vi "JL_Cycle_History_ParseRecord.vi"(5 "Low Level Tries":u8=5, 7 "Error In":errorcluster, 8 "Cycle History ERD":T1={"ERD Number"=61790, "Data Type"=enum."string"} {"ERD Number" format="%.0x"}, 9 "GEA Inputs":T2={"Source"=228, "Destination"=36} {"Destination" format="%.0x"; "Source" format="%.0x"}, 10 "GEA2 Reference In":refnum<k24>) -> (0 "Error Out":errorcluster, 1 "Bits":i32, 2 "CS2 Dryer":string[](array[string]), 3 "GEA2 Reference Out":refnum<k24>)   [LabVIEW 2023]
uses:
  D:/Common/LabVIEW GEA2 Toolkit/source/GEA3 DLL Source/GeaCommunication.dll
  Common/LabVIEW GEA2 Toolkit/source/GEA3 DLL Source/GeaCommunication.dll
  Common/LabVIEW GEA2 Toolkit/GEA3/type defs/Source_Destination.ctl
  Common/LabVIEW GEA2 Toolkit/GEA3/type defs/ERD Read Data In.ctl
  Common/LabVIEW GEA2 Toolkit/GEA3/library/GEA2_Toolkit.lvlib
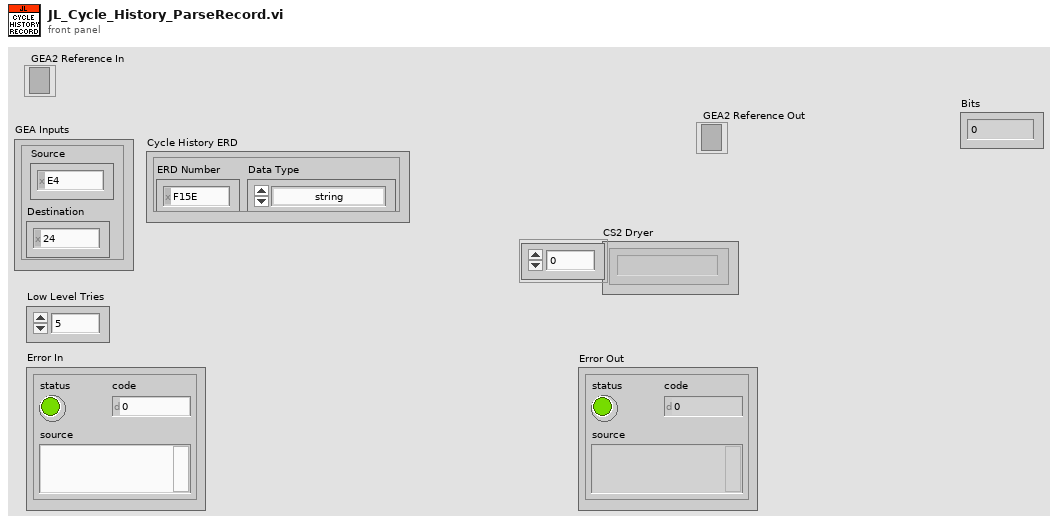
[diagram p1: front panel]
types:
  T1 = typedef "ERD Read Data In.ctl" = cluster{"ERD Number":u16, "Data Type":enum16{"string", "boolean", "uint8_t", "uint16_t", "uint32_t", "uint64_t", "int8_t", "int16_t", "int32_t", "int64_t"}}
  T2 = typedef "Source_Destination.ctl" = cluster{"Source":u8, "Destination":u8}
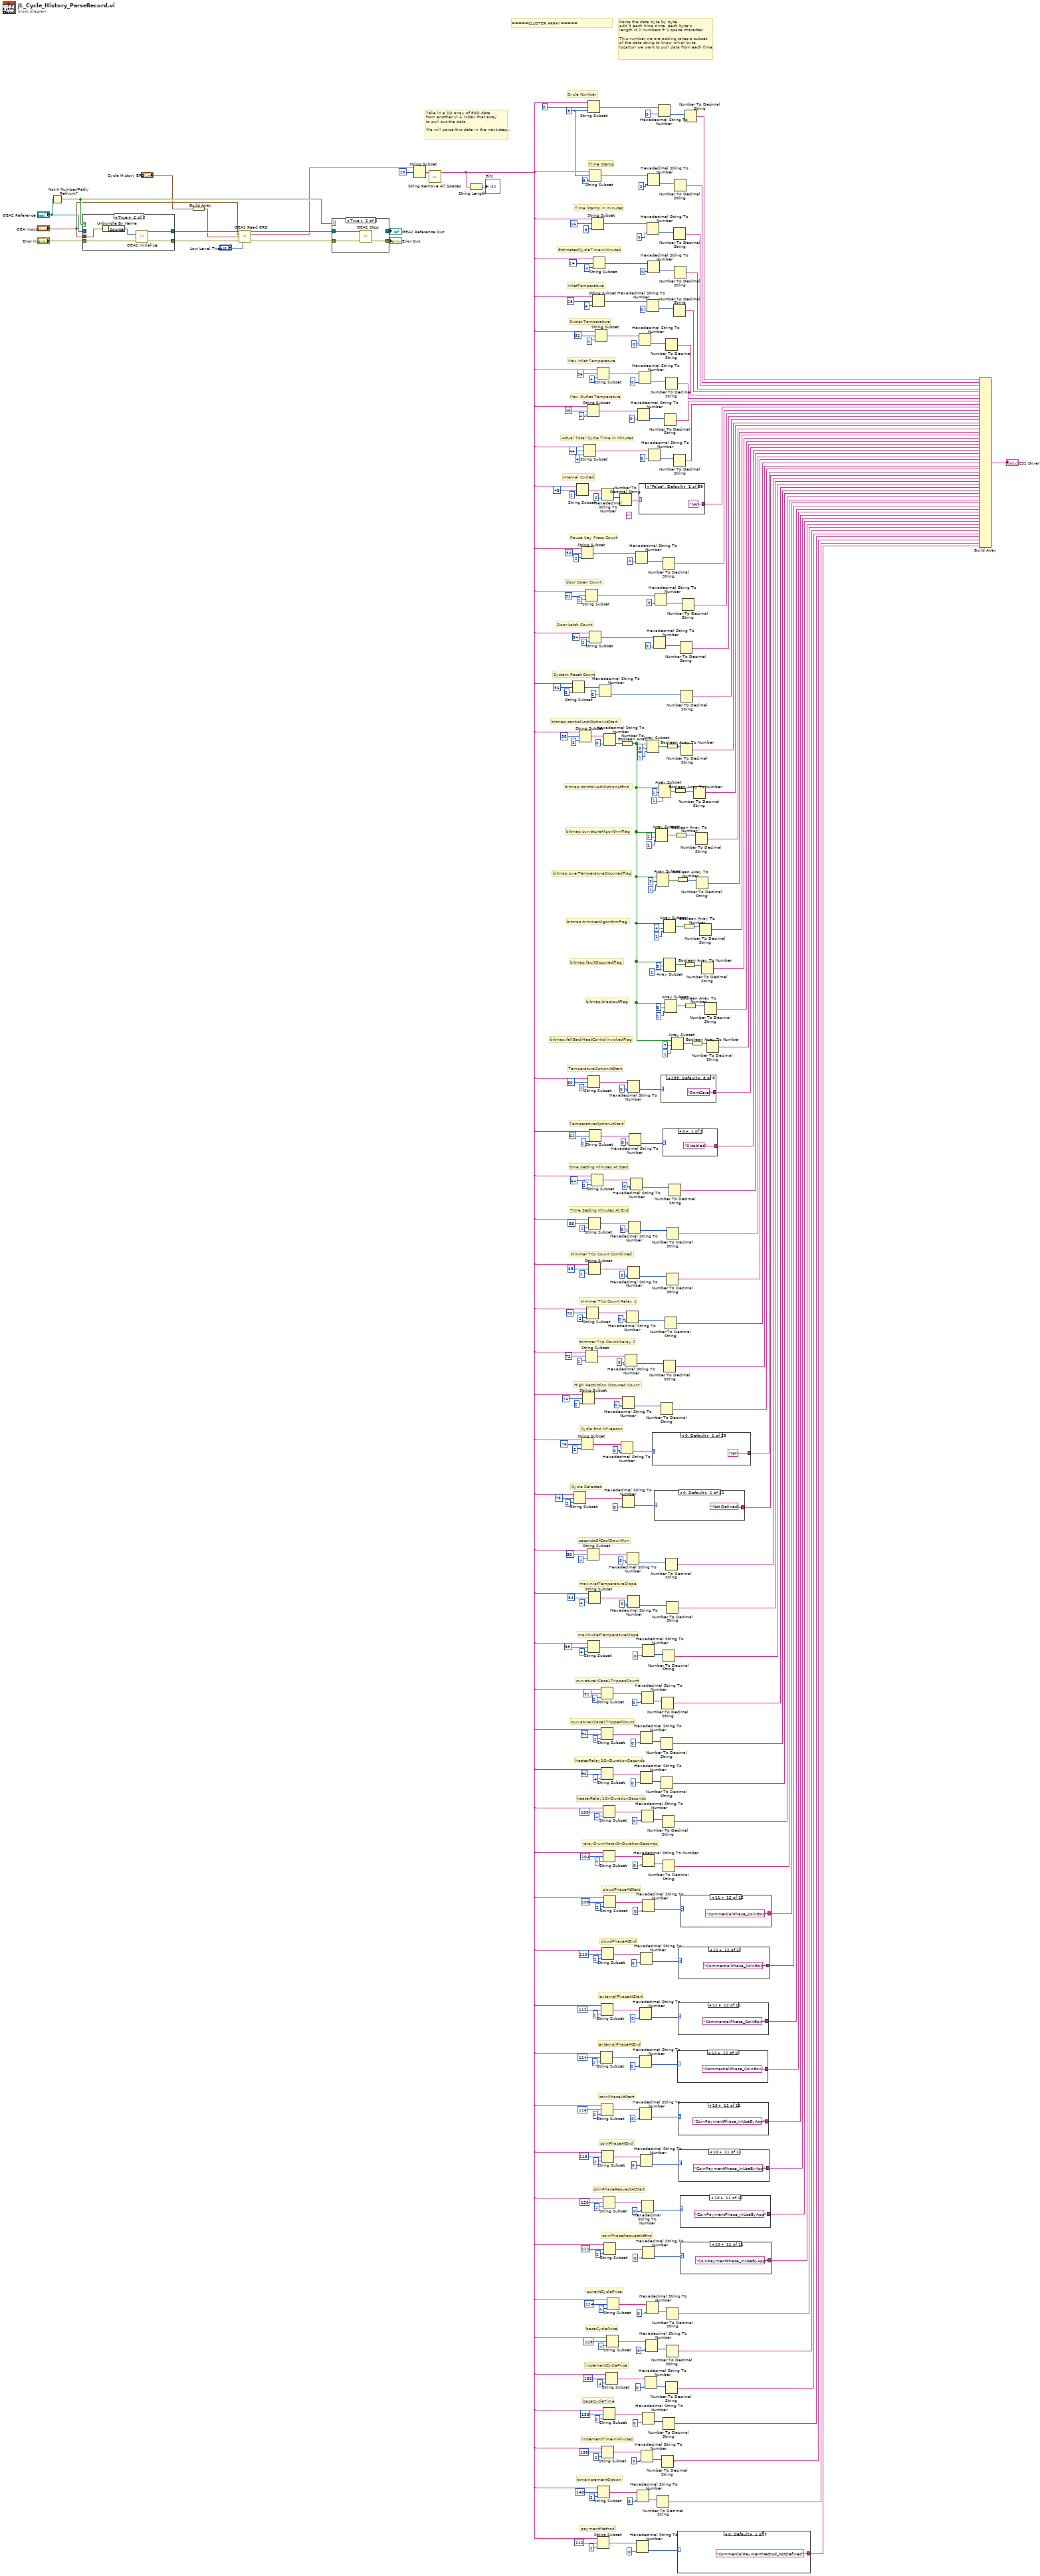
[diagram p0: block diagram]
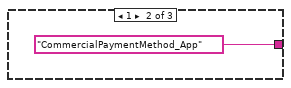
[diagram p2: hidden frame]
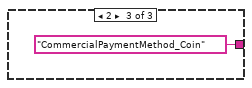
[diagram p3: hidden frame]
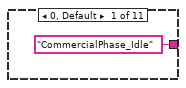
[diagram p4: hidden frame]
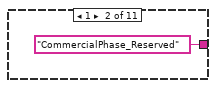
[diagram p5: hidden frame]
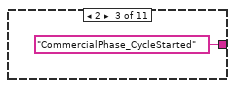
[diagram p6: hidden frame]
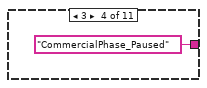
[diagram p7: hidden frame]
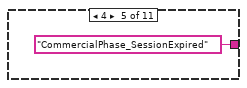
[diagram p8: hidden frame]
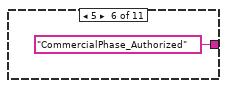
[diagram p9: hidden frame]
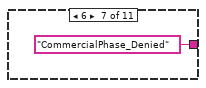
[diagram p10: hidden frame]
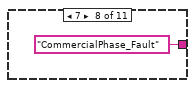
[diagram p11: hidden frame]
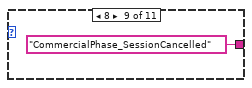
[diagram p12: hidden frame]
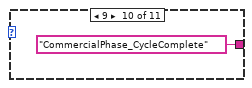
[diagram p13: hidden frame]
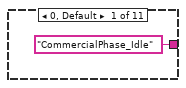
[diagram p14: hidden frame]
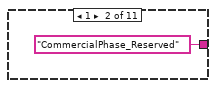
[diagram p15: hidden frame]
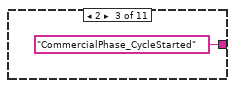
[diagram p16: hidden frame]
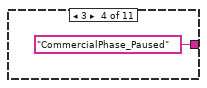
[diagram p17: hidden frame]
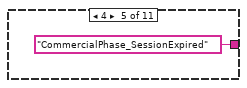
[diagram p18: hidden frame]
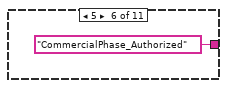
[diagram p19: hidden frame]
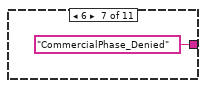
[diagram p20: hidden frame]
diagram:
  (unwired) ""
  w254 = 8 ("length (rest)")
  # "paymentMethod"
  # "timeIncrementOption"
  # "incrementTimeInMinutes"
  # "baseCycleTime"
  # "incrementCyclePrice"
  # "baseCyclePrice"
  # "currentCyclePrice"
  # "coinPhaseRequestAtEnd"
  # "coinPhaseRequestAtStart"
  # "coinPhaseAtEnd"
  # "coinPhaseAtStart"
  # "externalPhaseAtEnd"
  # "externalPhaseAtStart"
  # "cloudPhaseAtEnd"
  # "cloudPhaseAtStart"
  # "relayDrumMotorOnDurationSeconds"
  # "heaterRelay1OnDurationSeconds"
  # "heaterRelay1OnDurationSeconds"
  # "maxInletTemperatureSlope"
  # "secondsOfCoolDownRun"
  # "Cycle End Of reason"
  # "High Restriction Occurred Count"
  # "trimmer Trip Count Relay 2"
  # "trimmer Trip Count Relay 1"
  # "trimmer Trip Count Combined"
  # "Time Setting Minutes At End"
  # "time Setting Minutes At Start"
  # "TemperatureOptionAtStart"
  # "TemperatureOptionAtStart"
  # "bitmap.overTemperatureOccurredFlag"
  # "bitmap.curvatureAlgorithmFlag"
  # "bitmap.controlLockOptionAtEnd"
  # "Pause Key Press Count"
  # "InletTemperature"
  # "Take in a 1D array of ERD data\nfrom another VI & index that array\nto pull out the data. \n\nWe will parse this data in the next step..."
  # "Parse the data byte by byte...\nadd 3 each time since  each byte's\nlength is 2 numbers + 1 space character.\n\nThis number we are adding takes a subset\nof the data string to know which byte\nlocation we want to pull data from each time."
  # "=====CLUSTER ARRAY====="
  # "curvatureIICase1TrippedCount"
  # "curvatureIICase2TrippedCount"
  # "maxOutletTemperatureSlope"
  # "Cycle Selected"
  # "bitmap.fallBackHeatControlInvokedFlag"
  # "bitmap.blackoutFlag"
  # "bitmap.faultOccurredFlag"
  # "bitmap.trimmerAlgorithmFlag"
  # "bitmap.controlLockOptionAtStart"
  # "System Reset Count"
  # "Door Latch Count"
  # "door Open Count"
  # "Internal Cycled"
  # "Actual Total Cycle Time In Minutes"
  # "Max Outlet Temperature"
  # "Max Inlet Temperature"
  # "Outlet Temperature"
  # "EstimatedCycleTimeInMinutes"
  # "Time Stamp in minutes"
  # "Time Stamp"
  # "Cycle Number"
  n1 = Not A Number/Path/Refnum?(number/path/refnum="GEA2 Reference In") -> (NaN/Path/Refnum?=w326:bool)
  n2 = case shown="True" w326 {
    tunnel: "GEA Inputs" -> [_ w354]
    tunnel: "Error In" -> [w349 w353]
    tunnel: [w349 w352] -> w319
    tunnel: [w348 w351] -> w324
    tunnel: "GEA2 Reference In" -> [w348 _]
    frame False {
    }
    frame True {
      n3 = Unbundle By Name(w354) -> ("Source"=w350:u8)
      n4 = call "GEA2 Initialize.vi"("Source Address"=w350, "error in"=w353) -> ("GEA2 Reference Out"=w351:refnum<k24>, "error out"=w352:errorcluster)  [unwired: 10 in, 2 out]
    }
  }
  n5 = Build Array("Cycle History ERD") -> (w315:T1[])
  n6 = call "GEA2 Read ERD.vi"("GEA2 Reference In"=w324, "GEA Inputs"="GEA Inputs", "Read ERD List"=w315, "Error In"=w319, "Low Level Tries"="Low Level Tries") -> ("GEA2 Reference Out"=w322:refnum<k24>, "Raw Data Out"=w320:string, "Error Out"=w321:errorcluster)  [unwired: 7 in, 1 out]
  n7 = case shown="True" w326 {
    tunnel: [w355 w359] -> w327
    tunnel: [w356 _] -> w325
    tunnel: w322 -> [w356 w357]
    tunnel: w321 -> [w355 w358]
    frame False {
    }
    frame True {
      n8 = call "GEA2 Stop.vi"("GEA2 Reference In"=w357, "Error In"=w358) -> ("Error Out"=w359:errorcluster)  [unwired: 13 in]
    }
  }
  "Error Out" <- w327
  "GEA2 Reference Out" <- w325
  n9 = String Subset(string=w320, offset (0)=28) -> (substring=w313:string)  [unwired: 1 in]
  n10 = call "String Remove All Spaces.vi"("Input String"=w313) -> ("Spaces Removed"=w2:string)  [unwired: 13 in, 1 out]
  n11 = String Length(string=w2) -> (length=→"Bits":i32)
  n12 = String Subset(string=w2, offset (0)=56, length (rest)=2 ("length (rest)")) -> (substring=w227:string)
  n13 = String Subset(string=w2, offset (0)=78, length (rest)=2 ("length (rest)")) -> (substring=w266:string)
  n14 = String Subset(string=w2, offset (0)=48, length (rest)=2 ("length (rest)")) -> (substring=w238:string)
  n15 = String Subset(string=w2, offset (0)=58, length (rest)=2 ("length (rest)")) -> (substring=w226:string)
  n16 = String Subset(string=w2, offset (0)=50, length (rest)=2 ("length (rest)")) -> (substring=w234:string)
  n17 = String Subset(string=w2, offset (0)=76, length (rest)=2 ("length (rest)")) -> (substring=w171:string)
  n18 = String Subset(string=w2, offset (0)=74, length (rest)=2 ("length (rest)")) -> (substring=w173:string)
  n19 = String Subset(string=w2, offset (0)=44, length (rest)=4 ("length (rest)")) -> (substring=w240:string)
  n20 = String Subset(string=w2, offset (0)=72, length (rest)=2 ("length (rest)")) -> (substring=w182:string)
  n21 = String Subset(string=w2, offset (0)=52, length (rest)=2 ("length (rest)")) -> (substring=w232:string)
  n22 = String Subset(string=w2, offset (0)=70, length (rest)=2 ("length (rest)")) -> (substring=w187:string)
  n23 = String Subset(string=w2, offset (0)=40, length (rest)=4 ("length (rest)")) -> (substring=w242:string)
  n24 = String Subset(string=w2, offset (0)=80, length (rest)=4 ("length (rest)")) -> (substring=w158:string)
  n25 = String Subset(string=w2, offset (0)=0, length (rest)=w254) -> (substring=w255:string)
  n26 = String Subset(string=w2, offset (0)=60, length (rest)=2 ("length (rest)")) -> (substring=w218:string)
  n27 = String Subset(string=w2, offset (0)=88, length (rest)=4 ("length (rest)")) -> (substring=w263:string)
  n28 = String Subset(string=w2, offset (0)=68, length (rest)=2 ("length (rest)")) -> (substring=w193:string)
  n29 = String Subset(string=w2, offset (0)=84, length (rest)=4 ("length (rest)")) -> (substring=w156:string)
  n30 = String Subset(string=w2, offset (0)=66, length (rest)=2 ("length (rest)")) -> (substring=w199:string)
  n31 = String Subset(string=w2, offset (0)=w254, length (rest)=8 ("length (rest)")) -> (substring=w253:string)
  n32 = String Subset(string=w2, offset (0)=54, length (rest)=2 ("length (rest)")) -> (substring=w230:string)
  n33 = String Subset(string=w2, offset (0)=62, length (rest)=2 ("length (rest)")) -> (substring=w210:string)
  n34 = String Subset(string=w2, offset (0)=64, length (rest)=2 ("length (rest)")) -> (substring=w205:string)
  n35 = String Subset(string=w2, offset (0)=16, length (rest)=8 ("length (rest)")) -> (substring=w252:string)
  n36 = String Subset(string=w2, offset (0)=28, length (rest)=4 ("length (rest)")) -> (substring=w248:string)
  n37 = String Subset(string=w2, offset (0)=24, length (rest)=4 ("length (rest)")) -> (substring=w250:string)
  n38 = String Subset(string=w2, offset (0)=32, length (rest)=4 ("length (rest)")) -> (substring=w246:string)
  n39 = String Subset(string=w2, offset (0)=36, length (rest)=4 ("length (rest)")) -> (substring=w244:string)
  n40 = String Subset(string=w2, offset (0)=142, length (rest)=2 ("length (rest)")) -> (substring=w40:string)
  n41 = String Subset(string=w2, offset (0)=140, length (rest)=2 ("length (rest)")) -> (substring=w45:string)
  n42 = Hexadecimal String To Number(string=w227, default (0uL)=u16 0) -> (number=w274:u16)  [unwired: 1 in, 1 out]
  n43 = String Subset(string=w2, offset (0)=114, length (rest)=2 ("length (rest)")) -> (substring=w106:string)
  n44 = String Subset(string=w2, offset (0)=92, length (rest)=2 ("length (rest)")) -> (substring=w260:string)
  n45 = String Subset(string=w2, offset (0)=112, length (rest)=2 ("length (rest)")) -> (substring=w112:string)
  n46 = String Subset(string=w2, offset (0)=116, length (rest)=2 ("length (rest)")) -> (substring=w100:string)
  n47 = String Subset(string=w2, offset (0)=94, length (rest)=2 ("length (rest)")) -> (substring=w257:string)
  n48 = String Subset(string=w2, offset (0)=96, length (rest)=4 ("length (rest)")) -> (substring=w143:string)
  n49 = String Subset(string=w2, offset (0)=110, length (rest)=2 ("length (rest)")) -> (substring=w118:string)
  n50 = String Subset(string=w2, offset (0)=118, length (rest)=2 ("length (rest)")) -> (substring=w94:string)
  n51 = Hexadecimal String To Number(string=w238, default (0uL)=u32 0) -> (number=w285:u32)  [unwired: 1 in, 1 out]
  n52 = String Subset(string=w2, offset (0)=138, length (rest)=2 ("length (rest)")) -> (substring=w51:string)
  n53 = String Subset(string=w2, offset (0)=100, length (rest)=4 ("length (rest)")) -> (substring=w135:string)
  n54 = String Subset(string=w2, offset (0)=120, length (rest)=2 ("length (rest)")) -> (substring=w83:string)
  n55 = String Subset(string=w2, offset (0)=104, length (rest)=4 ("length (rest)")) -> (substring=w131:string)
  n56 = String Subset(string=w2, offset (0)=136, length (rest)=2 ("length (rest)")) -> (substring=w59:string)
  n57 = Hexadecimal String To Number(string=w226, default (0uL)=u16 0) -> (number=w33:u16)  [unwired: 1 in, 1 out]
  n58 = String Subset(string=w2, offset (0)=108, length (rest)=2 ("length (rest)")) -> (substring=w124:string)
  n59 = String Subset(string=w2, offset (0)=122, length (rest)=2 ("length (rest)")) -> (substring=w88:string)
  n60 = String Subset(string=w2, offset (0)=132, length (rest)=4 ("length (rest)")) -> (substring=w65:string)
  n61 = String Subset(string=w2, offset (0)=128, length (rest)=4 ("length (rest)")) -> (substring=w69:string)
  n62 = String Subset(string=w2, offset (0)=124, length (rest)=4 ("length (rest)")) -> (substring=w77:string)
  n63 = Number To Decimal String(number=w285) -> (decimal integer string=w236:string)  [unwired: 1 in]
  n64 = Hexadecimal String To Number(string=w171, default (0uL)=u8 0) -> (number=w167:u8)  [unwired: 1 in, 1 out]
  n65 = Number To Boolean Array(number=w33) -> (Boolean array=w3:bool[])
  n66 = Hexadecimal String To Number(string=w266, default (0uL)=u32 0) -> (number=w164:u32)  [unwired: 1 in, 1 out]
  n67 = Hexadecimal String To Number(string=w173, default (0uL)=u32 0) -> (number=w177:u32)  [unwired: 1 in, 1 out]
  n68 = Hexadecimal String To Number(string=w182, default (0uL)=u8 0) -> (number=w180:u8)  [unwired: 1 in, 1 out]
  n69 = Hexadecimal String To Number(string=w187, default (0uL)=u32 0) -> (number=w189:u32)  [unwired: 1 in, 1 out]
  n70 = Hexadecimal String To Number(string=w158, default (0uL)=u32 0) -> (number=w162:u32)  [unwired: 1 in, 1 out]
  n71 = Hexadecimal String To Number(string=w218, default (0uL)=u32 0) -> (number=w215:u32)  [unwired: 1 in, 1 out]
  n72 = Hexadecimal String To Number(string=w193, default (0uL)=u32 0) -> (number=w191:u32)  [unwired: 1 in, 1 out]
  n73 = Hexadecimal String To Number(string=w156, default (0uL)=u8 0) -> (number=w152:u8)  [unwired: 1 in, 1 out]
  n74 = Hexadecimal String To Number(string=w199, default (0uL)=u32 0) -> (number=w201:u32)  [unwired: 1 in, 1 out]
  n75 = Hexadecimal String To Number(string=w210, default (0uL)=u32 0) -> (number=w213:u32)  [unwired: 1 in, 1 out]
  n76 = Hexadecimal String To Number(string=w205, default (0uL)=u32 0) -> (number=w203:u32)  [unwired: 1 in, 1 out]
  n77 = Hexadecimal String To Number(string=w234, default (0uL)=u16 0) -> (number=w282:u16)  [unwired: 1 in, 1 out]
  n78 = Hexadecimal String To Number(string=w40, default (0uL)=u8 0) -> (number=w38:u8)  [unwired: 1 in, 1 out]
  n79 = Hexadecimal String To Number(string=w45, default (0uL)=u8 0) -> (number=w46:u8)  [unwired: 1 in, 1 out]
  n80 = Hexadecimal String To Number(string=w242, default (0uL)=u32 0) -> (number=w291:u32)  [unwired: 1 in, 1 out]
  n81 = Hexadecimal String To Number(string=w246, default (0uL)=u32 0) -> (number=w297:u32)  [unwired: 1 in, 1 out]
  n82 = Hexadecimal String To Number(string=w244, default (0uL)=u32 0) -> (number=w293:u32)  [unwired: 1 in, 1 out]
  n83 = case shown="\"False\", Default" w236 {
    tunnel: ["NA" "Unmapped" "MixedLoad" "Casuals" "Delicates" "SpeedDry" "Jeans" "TimedDry" "WarmUp" "AirFluff" "SteamDewrinkle" "SteamRefresh" "SanitizeDry" "BulkyItems" "TowelsSheets" "Cottons" "CasualsLessDry" "CasualsMoreDry" "CottonsLessDry" "CottonsOptimumDry" "CottonsMoreDry" "DelicatesLessDry" "DelicatesMoreDry" "TimedDry1" "TimedDry2" "TimedDry3" "TimedDry4" "TimedDry5" "TimedDry6" "ActiveWear" "DeWrinkle" "EnergySaver" "WasherLink" "BlockedVent" "SmartVent" "Scent" "Max" "Downloaded"] -> w235
    frame "False", Default {
    }
    frame "0" {
    }
    frame "1" {
    }
    frame "2" {
    }
    frame "3" {
    }
    frame "4" {
    }
    frame "5" {
    }
    frame "6" {
    }
    frame "7" {
    }
    frame "8" {
    }
    frame "9" {
    }
    frame "10" {
    }
    frame "11" {
    }
    frame "12" {
    }
    frame "13" {
    }
    frame "14" {
    }
    frame "15" {
    }
    frame "16" {
    }
    frame "17" {
    }
    frame "18" {
    }
    frame "19" {
    }
    frame "20" {
    }
    frame "21" {
    }
    frame "22" {
    }
    frame "23" {
    }
    frame "24" {
    }
    frame "25" {
    }
    frame "26" {
    }
    frame "27" {
    }
    frame "28" {
    }
    frame "29" {
    }
    frame "30" {
    }
    frame "31" {
    }
    frame "32" {
    }
    frame "33" {
    }
    frame "34" {
    }
    frame "35" {
    }
    frame "36" {
    }
  }
  n84 = Hexadecimal String To Number(string=w106, default (0uL)=u8 0) -> (number=w108:u8)  [unwired: 1 in, 1 out]
  n85 = Hexadecimal String To Number(string=w112, default (0uL)=u8 0) -> (number=w110:u8)  [unwired: 1 in, 1 out]
  n86 = Hexadecimal String To Number(string=w100, default (0uL)=u8 0) -> (number=w98:u8)  [unwired: 1 in, 1 out]
  n87 = Hexadecimal String To Number(string=w257, default (0uL)=u32 0) -> (number=w258:u32)  [unwired: 1 in, 1 out]
  n88 = Hexadecimal String To Number(string=w143, default (0uL)=u32 0) -> (number=w142:u32)  [unwired: 1 in, 1 out]
  n89 = Hexadecimal String To Number(string=w118, default (0uL)=u8 0) -> (number=w120:u8)  [unwired: 1 in, 1 out]
  n90 = Hexadecimal String To Number(string=w94, default (0uL)=u8 0) -> (number=w96:u8)  [unwired: 1 in, 1 out]
  n91 = Hexadecimal String To Number(string=w51, default (0uL)=u32 0) -> (number=w52:u32)  [unwired: 1 in, 1 out]
  n92 = Hexadecimal String To Number(string=w260, default (0uL)=u32 0) -> (number=w262:u32)  [unwired: 1 in, 1 out]
  n93 = Hexadecimal String To Number(string=w135, default (0uL)=u32 0) -> (number=w136:u32)  [unwired: 1 in, 1 out]
  n94 = Hexadecimal String To Number(string=w83, default (0uL)=u8 0) -> (number=w85:u8)  [unwired: 1 in, 1 out]
  n95 = Hexadecimal String To Number(string=w131, default (0uL)=u32 0) -> (number=w130:u32)  [unwired: 1 in, 1 out]
  n96 = Hexadecimal String To Number(string=w59, default (0uL)=u8 0) -> (number=w58:u8)  [unwired: 1 in, 1 out]
  n97 = Hexadecimal String To Number(string=w263, default (0uL)=u32 0) -> (number=w264:u32)  [unwired: 1 in, 1 out]
  n98 = Hexadecimal String To Number(string=w124, default (0uL)=u8 0) -> (number=w122:u8)  [unwired: 1 in, 1 out]
  n99 = Hexadecimal String To Number(string=w88, default (0uL)=u8 0) -> (number=w86:u8)  [unwired: 1 in, 1 out]
  n100 = Hexadecimal String To Number(string=w65, default (0uL)=u32 0) -> (number=w64:u32)  [unwired: 1 in, 1 out]
  n101 = Hexadecimal String To Number(string=w69, default (0uL)=u32 0) -> (number=w70:u32)  [unwired: 1 in, 1 out]
  n102 = Hexadecimal String To Number(string=w77, default (0uL)=u32 0) -> (number=w76:u32)  [unwired: 1 in, 1 out]
  n103 = Array Subset(array=w3, index=0, length=1) -> (w34:bool[])
  n104 = Hexadecimal String To Number(string=w252, default (0uL)=u32 0) -> (number=w308:u32)  [unwired: 1 in, 1 out]
  n105 = Hexadecimal String To Number(string=w248, default (0uL)=u32 0) -> (number=w299:u32)  [unwired: 1 in, 1 out]
  n106 = Hexadecimal String To Number(string=w253, default (0uL)=u32 0) -> (number=w310:u32)  [unwired: 1 in, 1 out]
  n107 = Hexadecimal String To Number(string=w250, default (0uL)=u32 0) -> (number=w306:u32)  [unwired: 1 in, 1 out]
  n108 = Hexadecimal String To Number(string=w240, default (0uL)=u32 0) -> (number=w287:u32)  [unwired: 1 in, 1 out]
  n109 = case shown="0, Default" w167 {
    tunnel: ["NA" "EmptyDrum" "DryLoad" "CoolDownPaused" "xtendedTumblePaused" "KnobChange" "PowerButtonPressed" "CycleComplete" "EventSequenceCommunicationIssue" "CriticalFault" "RemoteStop" "ExtremeHeatDetected" "NonPausableCyclePaused" "SafetyCriticalWatchdogTimeout" "DontCare"] -> w166
    frame 0, Default {
    }
    frame 1 {
    }
    frame 2 {
    }
    frame 3 {
    }
    frame 4 {
    }
    frame 5 {
    }
    frame 6 {
    }
    frame 7 {
    }
    frame 8 {
    }
    frame 9 {
    }
    frame 10 {
    }
    frame 11 {
    }
    frame 12 {
    }
    frame 13 {
    }
    frame 14 {
    }
  }
  n110 = Hexadecimal String To Number(string=w230, default (0uL)=u16 0) -> (number=w276:u16)  [unwired: 1 in, 1 out]
  n111 = case shown="0, Default" w164 {
    tunnel: ["Not Defined" "Bulky Items" "Sanitize" "Towels/Sheets" "Mixed Load" "Jeans" "Delicates" "Cottons" "Easy Care" "Active Wear" "Timed Dry" "DeWrinkle" "Quick/Air Fluff" "Steam Refresh" "Steam Dewrinkle" "Speed Dry" "Mixed" "Quick dry" "Casuals" "Warm up" "Energy Saver"] -> w163
    frame 0, Default {
    }
    frame 4 {
    }
    frame 5 {
    }
    frame 6 {
    }
    frame 8 {
    }
    frame 11 {
    }
    frame 13 {
    }
    frame 128 {
    }
    frame 129 {
    }
    frame 130 {
    }
    frame 131 {
    }
    frame 132 {
    }
    frame 133 {
    }
    frame 134 {
    }
    frame 135 {
    }
    frame 136 {
    }
    frame 137 {
    }
    frame 138 {
    }
    frame 139 {
    }
    frame 140 {
    }
    frame 141 {
    }
  }
  n112 = Hexadecimal String To Number(string=w232, default (0uL)=u16 0) -> (number=w280:u16)  [unwired: 1 in, 1 out]
  n113 = Array Subset(array=w3, index=2, length=1) -> (w25:bool[])
  n114 = Array Subset(array=w3, index=3, length=1) -> (w21:bool[])
  n115 = Number To Decimal String(number=w46) -> (decimal integer string=w43:string)  [unwired: 1 in]
  n116 = Hexadecimal String To Number(string=w255, default (0uL)=u32 0) -> (number=w312:u32)  [unwired: 1 in, 1 out]
  n117 = Array Subset(array=w3, index=1, length=1) -> (w29:bool[])
  n118 = Number To Decimal String(number=w258) -> (decimal integer string=w145:string)  [unwired: 1 in]
  n119 = Number To Decimal String(number=w142) -> (decimal integer string=w139:string)  [unwired: 1 in]
  n120 = case shown="255, Default" w215 {
    tunnel: ["Disabled" "NoHeat" "ExtraLow" "Low" "Medium" "High" "Max" "DontCare"] -> w214
    frame 0 {
    }
    frame 1 {
    }
    frame 2 {
    }
    frame 3 {
    }
    frame 4 {
    }
    frame 5 {
    }
    frame 6 {
    }
    frame 255, Default {
    }
  }
  n121 = Number To Decimal String(number=w177) -> (decimal integer string=w172:string)  [unwired: 1 in]
  n122 = Number To Decimal String(number=w52) -> (decimal integer string=w49:string)  [unwired: 1 in]
  n123 = Number To Decimal String(number=w262) -> (decimal integer string=w146:string)  [unwired: 1 in]
  n124 = Number To Decimal String(number=w136) -> (decimal integer string=w133:string)  [unwired: 1 in]
  n125 = Number To Decimal String(number=w282) -> (decimal integer string=w281:string)  [unwired: 1 in]
  n126 = case shown="0" w213 {
    tunnel: ["Disabled" "NoHeat" "ExtraLow" "Low" "Medium" "High" "Max" "DontCare"] -> w208
    frame 0 {
    }
    frame 1 {
    }
    frame 2 {
    }
    frame 3 {
    }
    frame 4 {
    }
    frame 5 {
    }
    frame 6 {
    }
    frame 255, Default {
    }
  }
  n127 = Number To Decimal String(number=w130) -> (decimal integer string=w127:string)  [unwired: 1 in]
  n128 = Number To Decimal String(number=w58) -> (decimal integer string=w55:string)  [unwired: 1 in]
  n129 = Number To Decimal String(number=w264) -> (decimal integer string=w149:string)  [unwired: 1 in]
  n130 = Array Subset(array=w3, index=4, length=1) -> (w17:bool[])
  n131 = Array Subset(array=w3, index=5, length=1) -> (w13:bool[])
  n132 = Number To Decimal String(number=w180) -> (decimal integer string=w178:string)  [unwired: 1 in]
  n133 = Number To Decimal String(number=w291) -> (decimal integer string=w289:string)  [unwired: 1 in]
  n134 = Array Subset(array=w3, index=6, length=1) -> (w9:bool[])
  n135 = Number To Decimal String(number=w189) -> (decimal integer string=w179:string)  [unwired: 1 in]
  n136 = Number To Decimal String(number=w297) -> (decimal integer string=w295:string)  [unwired: 1 in]
  n137 = Number To Decimal String(number=w293) -> (decimal integer string=w292:string)  [unwired: 1 in]
  n138 = Number To Decimal String(number=w162) -> (decimal integer string=w157:string)  [unwired: 1 in]
  n139 = Number To Decimal String(number=w64) -> (decimal integer string=w61:string)  [unwired: 1 in]
  n140 = Number To Decimal String(number=w70) -> (decimal integer string=w67:string)  [unwired: 1 in]
  n141 = Boolean Array To Number(Boolean array=w34) -> (number=w32:u32)
  n142 = Number To Decimal String(number=w191) -> (decimal integer string=w190:string)  [unwired: 1 in]
  n143 = Number To Decimal String(number=w152) -> (decimal integer string=w151:string)  [unwired: 1 in]
  n144 = Number To Decimal String(number=w76) -> (decimal integer string=w73:string)  [unwired: 1 in]
  n145 = Number To Decimal String(number=w201) -> (decimal integer string=w196:string)  [unwired: 1 in]
  n146 = Number To Decimal String(number=w203) -> (decimal integer string=w202:string)  [unwired: 1 in]
  n147 = Array Subset(array=w3, index=7, length=1) -> (w5:bool[])
  n148 = Number To Decimal String(number=w308) -> (decimal integer string=w307:string)  [unwired: 1 in]
  n149 = Number To Decimal String(number=w299) -> (decimal integer string=w298:string)  [unwired: 1 in]
  n150 = Number To Decimal String(number=w287) -> (decimal integer string=w286:string)  [unwired: 1 in]
  n151 = Number To Decimal String(number=w310) -> (decimal integer string=w309:string)  [unwired: 1 in]
  n152 = Number To Decimal String(number=w306) -> (decimal integer string=w301:string)  [unwired: 1 in]
  n153 = Boolean Array To Number(Boolean array=w29) -> (number=w28:u32)
  n154 = Boolean Array To Number(Boolean array=w25) -> (number=w24:u32)
  n155 = Boolean Array To Number(Boolean array=w21) -> (number=w20:u32)
  n156 = case shown="0, Default" w38 {
    tunnel: ["CommercialPaymentMethod_NotDefined" "CommercialPaymentMethod_App" "CommercialPaymentMethod_Coin"] -> w37
    frame 0, Default {
    }
    frame 1 {
    }
    frame 2 {
    }
  }
  n157 = case shown="11" w108 {
    tunnel: ["CommercialPhase_Idle" "CommercialPhase_Reserved" "CommercialPhase_CycleRequested" "CommercialPhase_CycleStarted" "CommercialPhase_Paused" "CommercialPhase_SessionExpired" "CommercialPhase_Authorized" "CommercialPhase_Denied" "CommercialPhase_Fault" "CommercialPhase_SessionCancelled" "CommercialPhase_CycleComplete" "CommercialPhase_CoinBox"] -> w103
    frame 0, Default {
    }
    frame 1 {
    }
    frame 2 {
    }
    frame 3 {
    }
    frame 4 {
    }
    frame 5 {
    }
    frame 6 {
    }
    frame 7 {
    }
    frame 8 {
    }
    frame 9 {
    }
    frame 10 {
    }
    frame 11 {
    }
  }
  n158 = case shown="11" w110 {
    tunnel: ["CommercialPhase_Idle" "CommercialPhase_Reserved" "CommercialPhase_CycleRequested" "CommercialPhase_CycleStarted" "CommercialPhase_Paused" "CommercialPhase_SessionExpired" "CommercialPhase_Authorized" "CommercialPhase_Denied" "CommercialPhase_Fault" "CommercialPhase_SessionCancelled" "CommercialPhase_CycleComplete" "CommercialPhase_CoinBox"] -> w109
    frame 0, Default {
    }
    frame 1 {
    }
    frame 2 {
    }
    frame 3 {
    }
    frame 4 {
    }
    frame 5 {
    }
    frame 6 {
    }
    frame 7 {
    }
    frame 8 {
    }
    frame 9 {
    }
    frame 10 {
    }
    frame 11 {
    }
  }
  n159 = case shown="10" w98 {
    tunnel: ["CommercialPhase_Idle" "CommercialPhase_Reserved" "CommercialPhase_CycleStarted" "CommercialPhase_Paused" "CommercialPhase_SessionExpired" "CommercialPhase_Authorized" "CommercialPhase_Denied" "CommercialPhase_Fault" "CommercialPhase_SessionCancelled" "CommercialPhase_CycleComplete" "CoinPaymentPhase_InUseByApp"] -> w97
    frame 0, Default {
    }
    frame 1 {
    }
    frame 2 {
    }
    frame 3 {
    }
    frame 4 {
    }
    frame 5 {
    }
    frame 6 {
    }
    frame 7 {
    }
    frame 8 {
    }
    frame 9 {
    }
    frame 10 {
    }
  }
  n160 = case shown="11" w120 {
    tunnel: ["CommercialPhase_Idle" "CommercialPhase_Reserved" "CommercialPhase_CycleRequested" "CommercialPhase_CycleStarted" "CommercialPhase_Paused" "CommercialPhase_SessionExpired" "CommercialPhase_Authorized" "CommercialPhase_Denied" "CommercialPhase_Fault" "CommercialPhase_SessionCancelled" "CommercialPhase_CycleComplete" "CommercialPhase_CoinBox"] -> w115
    frame 0, Default {
    }
    frame 1 {
    }
    frame 2 {
    }
    frame 3 {
    }
    frame 4 {
    }
    frame 5 {
    }
    frame 6 {
    }
    frame 7 {
    }
    frame 8 {
    }
    frame 9 {
    }
    frame 10 {
    }
    frame 11 {
    }
  }
  n161 = case shown="10" w96 {
    tunnel: ["CommercialPhase_Idle" "CommercialPhase_Reserved" "CommercialPhase_CycleStarted" "CommercialPhase_Paused" "CommercialPhase_SessionExpired" "CommercialPhase_Authorized" "CommercialPhase_Denied" "CommercialPhase_Fault" "CommercialPhase_SessionCancelled" "CommercialPhase_CycleComplete" "CoinPaymentPhase_InUseByApp"] -> w91
    frame 0, Default {
    }
    frame 1 {
    }
    frame 2 {
    }
    frame 3 {
    }
    frame 4 {
    }
    frame 5 {
    }
    frame 6 {
    }
    frame 7 {
    }
    frame 8 {
    }
    frame 9 {
    }
    frame 10 {
    }
  }
  n162 = case shown="10" w85 {
    tunnel: ["CommercialPhase_Idle" "CommercialPhase_Reserved" "CommercialPhase_CycleStarted" "CommercialPhase_Paused" "CommercialPhase_SessionExpired" "CommercialPhase_Authorized" "CommercialPhase_Denied" "CommercialPhase_Fault" "CommercialPhase_SessionCancelled" "CommercialPhase_CycleComplete" "CoinPaymentPhase_InUseByApp"] -> w80
    frame 0, Default {
    }
    frame 1 {
    }
    frame 2 {
    }
    frame 3 {
    }
    frame 4 {
    }
    frame 5 {
    }
    frame 6 {
    }
    frame 7 {
    }
    frame 8 {
    }
    frame 9 {
    }
    frame 10 {
    }
  }
  n163 = Number To Decimal String(number=w276) -> (decimal integer string=w275:string)  [unwired: 1 in]
  n164 = case shown="11" w122 {
    tunnel: ["CommercialPhase_Idle" "CommercialPhase_Reserved" "CommercialPhase_CycleRequested" "CommercialPhase_CycleStarted" "CommercialPhase_Paused" "CommercialPhase_SessionExpired" "CommercialPhase_Authorized" "CommercialPhase_Denied" "CommercialPhase_Fault" "CommercialPhase_SessionCancelled" "CommercialPhase_CycleComplete" "CommercialPhase_CoinBox"] -> w121
    frame 0, Default {
    }
    frame 1 {
    }
    frame 2 {
    }
    frame 3 {
    }
    frame 4 {
    }
    frame 5 {
    }
    frame 6 {
    }
    frame 7 {
    }
    frame 8 {
    }
    frame 9 {
    }
    frame 10 {
    }
    frame 11 {
    }
  }
  n165 = case shown="10" w86 {
    tunnel: ["CommercialPhase_Idle" "CommercialPhase_Reserved" "CommercialPhase_CycleStarted" "CommercialPhase_Paused" "CommercialPhase_SessionExpired" "CommercialPhase_Authorized" "CommercialPhase_Denied" "CommercialPhase_Fault" "CommercialPhase_SessionCancelled" "CommercialPhase_CycleComplete" "CoinPaymentPhase_InUseByApp"] -> w79
    frame 0, Default {
    }
    frame 1 {
    }
    frame 2 {
    }
    frame 3 {
    }
    frame 4 {
    }
    frame 5 {
    }
    frame 6 {
    }
    frame 7 {
    }
    frame 8 {
    }
    frame 9 {
    }
    frame 10 {
    }
  }
  n166 = Number To Decimal String(number=w274) -> (decimal integer string=w271:string)  [unwired: 1 in]
  n167 = Number To Decimal String(number=w32) -> (decimal integer string=w270:string)  [unwired: 1 in]
  n168 = Number To Decimal String(number=w280) -> (decimal integer string=w278:string)  [unwired: 1 in]
  n169 = Boolean Array To Number(Boolean array=w17) -> (number=w16:u32)
  n170 = Boolean Array To Number(Boolean array=w13) -> (number=w12:u32)
  n171 = Boolean Array To Number(Boolean array=w9) -> (number=w8:u32)
  n172 = Number To Decimal String(number=w312) -> (decimal integer string=w311:string)  [unwired: 1 in]
  n173 = Boolean Array To Number(Boolean array=w5) -> (number=w4:u32)
  n174 = Number To Decimal String(number=w28) -> (decimal integer string=w269:string)  [unwired: 1 in]
  n175 = Number To Decimal String(number=w24) -> (decimal integer string=w268:string)  [unwired: 1 in]
  n176 = Number To Decimal String(number=w20) -> (decimal integer string=w224:string)  [unwired: 1 in]
  n177 = Number To Decimal String(number=w16) -> (decimal integer string=w223:string)  [unwired: 1 in]
  n178 = Number To Decimal String(number=w12) -> (decimal integer string=w222:string)  [unwired: 1 in]
  n179 = Number To Decimal String(number=w8) -> (decimal integer string=w221:string)  [unwired: 1 in]
  n180 = Number To Decimal String(number=w4) -> (decimal integer string=w220:string)  [unwired: 1 in]
  n181 = Build Array(w311, w309, w307, w301, w298, w295, w292, w289, w286, w235, w281, w278, w275, w271, w270, w269, w268, w224, w223, w222, w221, w220, w214, w208, w202, w196, w190, w179, w178, w172, w166, w163, w157, w151, w149, w146, w145, w139, w133, w127, w121, w115, w109, w103, w97, w91, w80, w79, w73, w67, w61, w55, w49, w43, w37) -> (→"CS2 Dryer":string[])
